vi "VI Tree - buttons.vi"   [LabVIEW 2009]
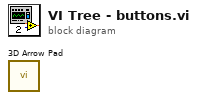
[diagram p0: block diagram]
diagram:
  n1 = call "3D Arrow Pad.vi"() -> ()  [unwired: 1 in]
